vi "LEP_RV_Check_uV4.vi"(8 "error in (no error)":errorcluster, 11 "KEIL Path":path) -> (0 "error out":errorcluster, 3 "uv4 installed":bool)   [LabVIEW 2011]
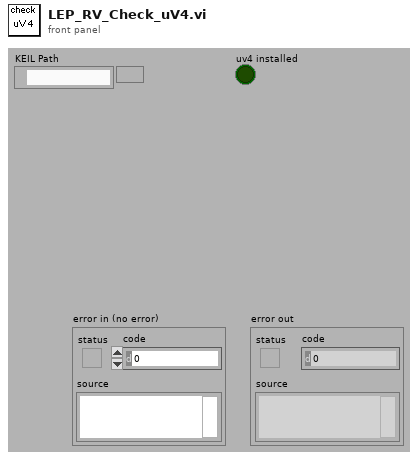
[diagram p1: front panel]
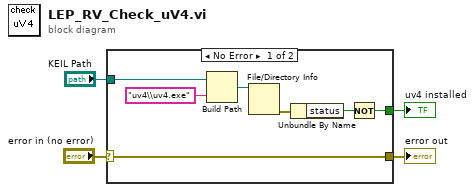
[diagram p0: block diagram]
diagram:
  n1 = case shown="No Error" "error in (no error)" {
    selector: "error in (no error)" -> [w6 w12]
    tunnel: [w6 w12] -> w3
    tunnel: [w7 _] -> w2
    tunnel: "KEIL Path" -> [w5 _]
    frame No Error {
      n2 = Build Path(base path=w5, name or relative path="uv4\\uv4.exe") -> (appended path=w10:path)
      n3 = File/Directory Info(path=w10) -> (error out=w9:errorcluster)  [unwired: 1 in, 6 out]
      n4 = Unbundle By Name(w9) -> ("status"=w8:bool)
      n5 = Not(x=w8) -> (.not. x?=w7:bool)
    }
    frame Error {
    }
  }
  "error out" <- w3
  "uv4 installed" <- w2
